vi "Manipulator PWM-y.vi"(4 "Boolean":bool, 6 "button in":bool, 7 "X axis":i32, 9 "button 1":bool, 10 "Z axis":i32, 11 "Y":i32) -> (2 "String":string)   [LabVIEW 2014]
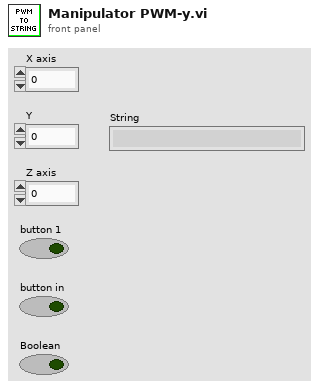
[diagram p1: front panel]
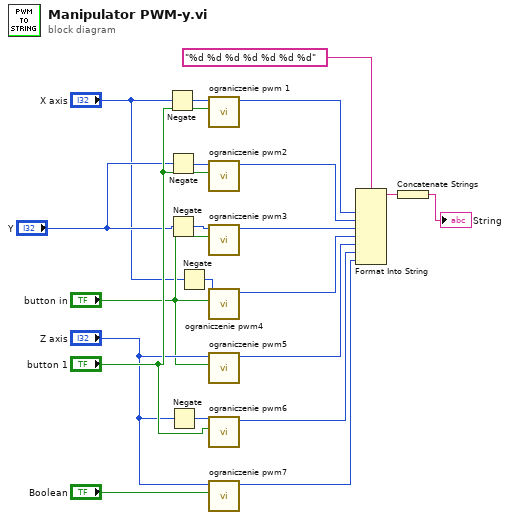
[diagram p0: block diagram]
diagram:
  n1 = Negate(x="X axis") -> (-x=w7:i32)
  n2 = Negate(x="Y") -> (-x=w6:i32)
  n3 = Negate(x="Y") -> (-x=w5:i32)
  n4 = Negate(x="Z axis") -> (-x=w9:i32)
  n5 = Negate(x="X axis") -> (-x=w2:i32)
  n6 = call "ograniczenie pwm 1.vi"("button 1"="button 1", "X axis"=w7) -> ("y"=w18:i16)  [unwired: 9 in]
  n7 = call "ograniczenie pwm2.vi"("button 1"="button 1", "X axis"=w6) -> ("y"=w19:i16)  [unwired: 9 in]
  n8 = call "ograniczenie pwm3.vi"("button 1"="button in", "X axis"=w5) -> ("y"=w13:i16)  [unwired: 9 in]
  n9 = call "ograniczenie pwm4.vi"("button 1"="button in", "X axis"=w2) -> ("y"=w14:i16)  [unwired: 9 in]
  n10 = call "ograniczenie pwm5.vi"("button 1"="button in", "X axis"="Z axis") -> ("y"=w16:i16)  [unwired: 9 in]
  n11 = call "ograniczenie pwm6.vi"("button 1"="button 1", "X axis"=w9) -> ("y"=w15:i16)  [unwired: 9 in]
  n12 = call "ograniczenie pwm7.vi"("button 1"="Boolean", "X axis"="Z axis") -> ("y"=w17:i16)  [unwired: 9 in]
  n13 = Format Into String(format string="%d %d %d %d %d %d %d", w18, w19, w13, w14, w16, w15, w17) -> (resulting string=w12:string)  [unwired: 2 in, 1 out]
  n14 = Concatenate Strings(w12) -> (→"String":string)
